vi "Inatke Controller.vi"(8 "error in":errorcluster) -> ()   [LabVIEW 2023]
doc: "This VI executes continuously carrying out the current operation and responding to updates or new operations. It will often contain the timing or control code that is difficult to place directly in TeleOp. This VI generally opens all sensors and motors and isolates the rest of the robot code from knowing how the operations are carried out."
uses:
  <vilib>/Rock Robotics/WPI/Framework/Completion Status.ctl
  Inatke Setpoints.ctl
  <vilib>/Rock Robotics/WPI/Solenoid/WPI_SolenoidValue.ctl
  Transfer/Implementation/Transfer Setpoints.ctl
  Transfer/Implementation/Transfer Operations.ctl
  <vilib>/Rock Robotics/WPI/Solenoid/WPI_SolenoidSetEnum.vi
  Framework/Robot Global Data.vi
  <vilib>/Rock Robotics/Network Tables/NT Write Boolean.vi
panel:
  in  "Bottom":dbl=0.62 format="%#_13g"
  in  "top":dbl=0.52 format="%#_13g"
  in  "Interactive Values":T1
  out "Current\nCmd":string="Started at  09:43:49.164\nDefault: Reserve,  "
  in  "Buttons":cluster{"Execute Cmd":bool, "Abort Cmd":bool}
  out "Command Timing":cluster{"Start Time (ms)":u32, "Iterations":i32}={"Start Time (ms)"=7327, "Iterations"=0}
  out "Status":T2
  # "Tip: It may be helpful to observe inputs and sensor values.\nYou may also want to display tuning or debugging controls."
  # "Interactive Command: You may fill in the settings for a command\nand schedule it with the Execute button. You can observe and abort\nany command while fine tuning the code for the controller."
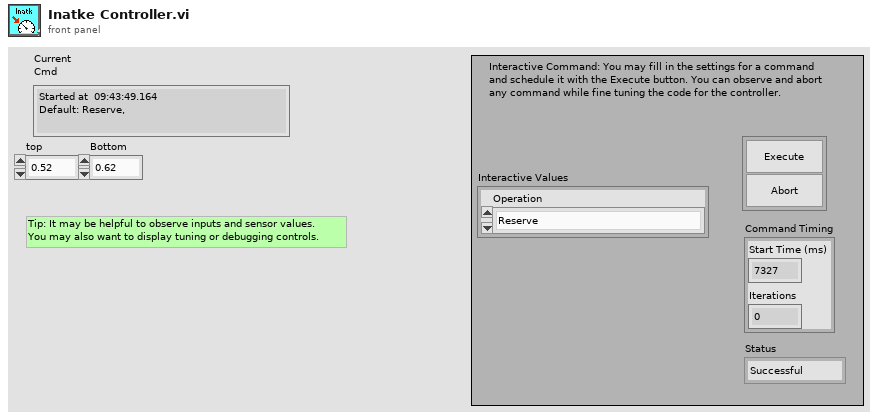
[diagram p1: front panel]
types:
  T1 = typedef "Inatke Setpoints.ctl" = cluster{"Operation":enum16{"Reserve", "Read Current", "Immediate", "Extend", "Retract", "Move Slow", "Reject"}}
  T2 = typedef "Completion Status.ctl" = enum16{"Successful", "Aborted", "Incomplete"}
  T3 = typedef "Command Status Info.ctl" = cluster{"Name":string, "Status":T2, "notifier out":T4}
  T4 = typedef "Completion Notifier.ctl" = refnum<notifier>
  T5 = cluster{"Current Command":T1, "Command Timing":cluster{"Start Time (ms)":u32, "Iterations":i32}, "Command Arguments":cluster{"Command Info":T3, "Description":string, "Default Command":T1, "queue out":refnum<queue>, "Subsystem Name":string}}
  T6 = typedef "WPI_SolenoidValue.ctl" = enum16{"Off", "On", "Forward", "Reverse"}
  T7 = typedef "Transfer Setpoints.ctl" = cluster{"Operation":T8}
  T8 = typedef "Transfer Operations.ctl" = enum16{"Reserve", "Read Current", "Immediate", "On", "Off", "Reject"}
  T9 = enum16{"Reserve", "Read Current", "Immediate", "Extend", "Retract", "Move Slow", "Reject"}
  T10 = typedef "WPI_MotorControlDeviceRef.ctl" = cluster{"DeviceStatus":errorcluster, "Type":T11, "PWM":cluster{"PWM Channel":T12, "DeadBand":T13}, "CAN":cluster{"Device Number":u8, "SetOutput VI Ref":variant, "GetOutput VI Ref":variant, "Enable VI Ref":variant, "Disable VI Ref":variant, "Data":variant}, "Invert":bool, "DIO PWM":cluster{"PWM \"Enable\" Channel":T12, "DIOChannel":T14, "PWM Rate":dbl}}
  T11 = typedef "WPI_MotorControlType.ctl" = enum16{"PWM", "CAN", "DIO PWM"}
  T12 = typedef "FPGA_DIOPWMChannel.ctl" = enum8{"PWM 0", "PWM 1", "PWM 2", "PWM 3", "PWM 4", "PWM 5", "PWM 6", "PWM 7", "PWM 8", "PWM 9", "PWM MXP 0", "PWM MXP 1", "PWM MXP 2", "PWM MXP 3", "PWM MXP 4", "PWM MXP 5", "PWM MXP 6", "PWM MXP 7", "PWM MXP 8", "PWM MXP 9", "Invalid"}
  T13 = typedef "WPI_PWMDeadband.ctl" = cluster{"Name":string, "maxPositivePwm":i32, "minPositivePwm":i32, "centerPwm":i32, "maxNegativePwm":i32, "minNegativePwm":i32, "angularRange":u16}
  T14 = typedef "FPGA_DIOChannel.ctl" = enum8{"DIO 0", "DIO 1", "DIO 2", "DIO 3", "DIO 4", "DIO 5", "DIO 6", "DIO 7", "DIO 8", "DIO 9", "DIO MXP 0", "DIO MXP 1", "DIO MXP 2", "DIO MXP 3", "DIO MXP 4", "DIO MXP 5", "DIO MXP 6", "DIO MXP 7", "DIO MXP 8", "DIO MXP 9", "DIO MXP 10", "DIO MXP 11", "DIO MXP 12", "DIO MXP 13", "DIO MXP 14", "DIO MXP 15", "SPI Port CS1", "SPI Port CS2", "SPI Port CS3", "SPI Port MISO", "SPI Port MOSI", "Invalid"}
  T15 = typedef "WPI_SolenoidDevRef.ctl" = cluster{"DevStatus":errorcluster, "Pneumatics Control Module":u8, "Forward Solenoid Channel":T16, "Reverse Solenoid Channel":T16}
  T16 = typedef "WPI_SolenoidChannel.ctl" = enum8{"Solenoid 0", "Solenoid 1", "Solenoid 2", "Solenoid 3", "Solenoid 4", "Solenoid 5", "Solenoid 6", "Solenoid 7", "Solenoid 8", "Solenoid 9", "Solenoid 10", "Solenoid 11", "Solenoid 12", "Solenoid 13", "Solenoid 14", "Solenoid 15", "Invalid"}
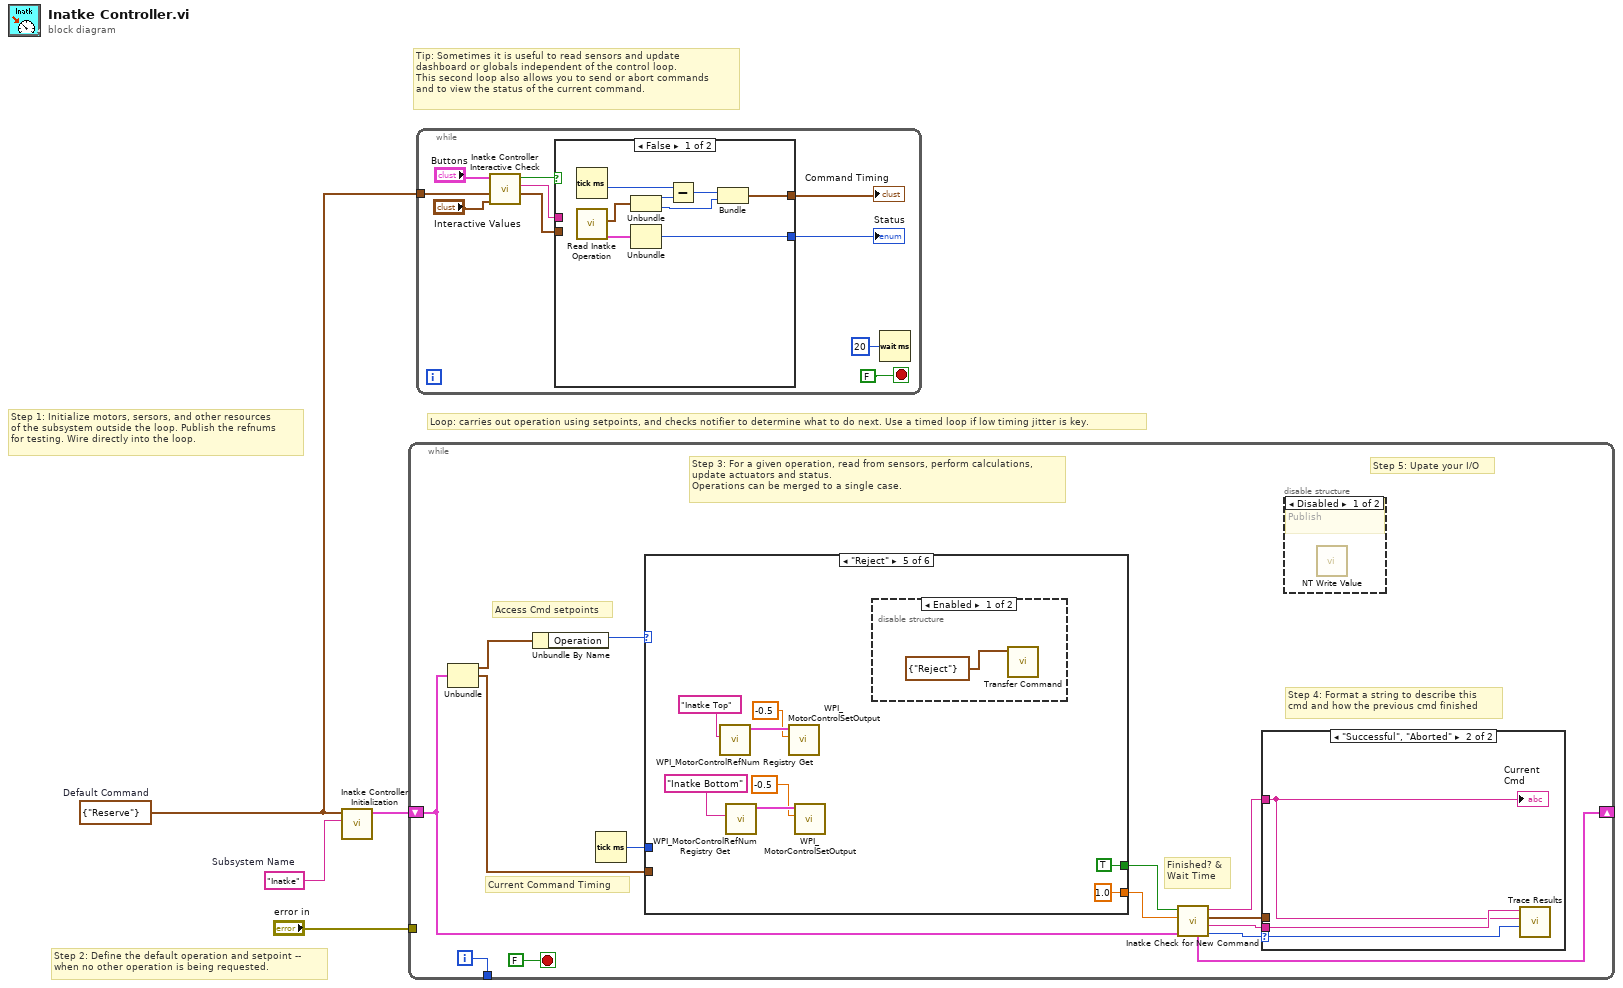
[diagram p0: block diagram]
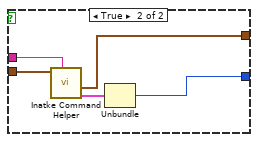
[diagram p2: hidden frame]
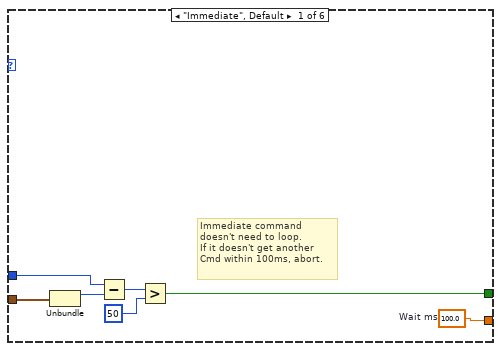
[diagram p5: hidden frame]
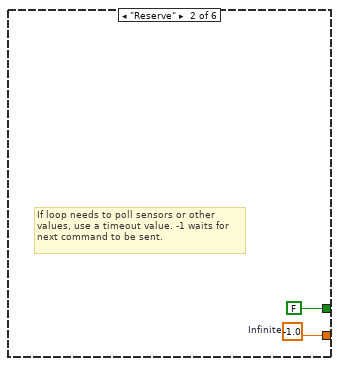
[diagram p6: hidden frame]
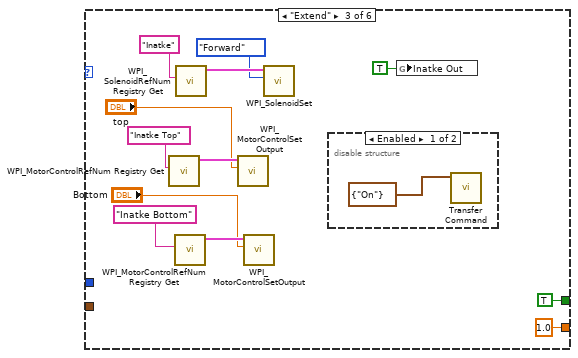
[diagram p7: hidden frame]
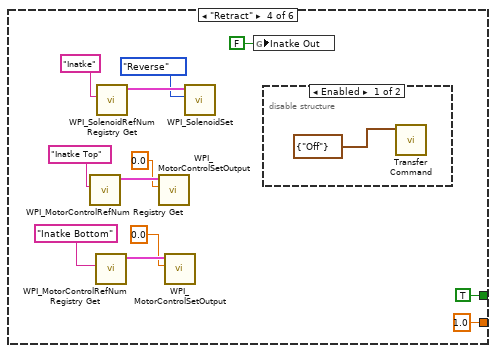
[diagram p9: hidden frame]
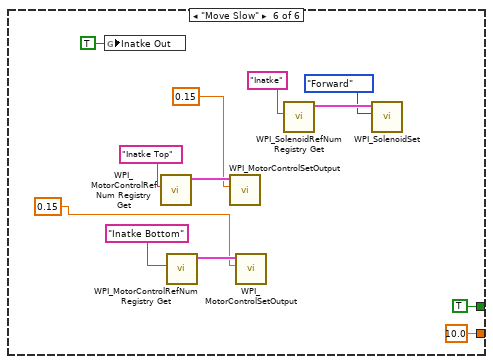
[diagram p12: hidden frame]
diagram:
  w1 = T1 {"Operation"=enum."Reserve"}  # Default Command
  w2 = "Inatke"  # Subsystem Name
  # "Tip: Sometimes it is useful to read sensors and update\ndashboard or globals independent of the control loop.\nThis second loop also allows you to send or abort commands\nand to view the status of the current command."
  # "Step 2: Define the default operation and setpoint --\nwhen no other operation is being requested."
  # "Step 1: Initialize motors, sersors, and other resources\nof the subsystem outside the loop. Publish the refnums\nfor testing. Wire directly into the loop."
  # "Loop: carries out operation using setpoints, and checks notifier to determine what to do next. Use a timed loop if low timing jitter is key."
  n1 = call "Inatke Controller Initialization.vi"("Subsystem Name"=w2, "Default Command"=w1) -> ("Current Command"=w3:T5)  [unwired: 9 in]
  n2 = while {
    shift-right: [w12] -> _
    shift-left: w3 -> [w5]
    tunnel: [w17] -> _
    tunnel: "error in" -> [_]
    i -> [w17]
    stop <- FALSE stop-if-true
    # "Step 5: Upate your I/O"
    # "Step 4: Format a string to describe this\ncmd and how the previous cmd finished"
    # "Current Command Timing"
    # "Access Cmd setpoints"
    # "Finished? &\nWait Time"
    # "Step 3: For a given operation, read from sensors, perform calculations,\nupdate actuators and status.\nOperations can be merged to a single case."
    n3 = Unbundle(w5) -> ("Current Command"=w16:T1, "Command Timing"=w13:cluster{"Start Time (ms)":u32, "Iterations":i32})  [unwired: 1 out]
    n4 = Unbundle By Name(w16) -> ("Operation"=w15:T9)
    n5 = Tick Count (ms)() -> (millisecond timer value=w14:u32)
    n6 = case shown="\"Reject\"" w15 {
      tunnel: [w28 w30 1.0 ("Infinite") 1.0 ("Infinite") 1.0 ("Infinite") 10.0 ("Infinite")] -> w10
      tunnel: [w22 FALSE ("ignore previous (F)") TRUE ("ignore previous (F)") TRUE ("ignore previous (F)") TRUE ("ignore previous (F)") TRUE ("ignore previous (F)")] -> w11
      tunnel: w13 -> [w24 _ _ _ _ _]
      tunnel: w14 -> [w23 _ _ _ _ _]
      frame "Immediate", Default {
        w28 = 100.0  # Wait ms
        # "Immediate command\ndoesn't need to loop.\nIf it doesn't get another\nCmd within 100ms, abort."
        n7 = Unbundle(w24) -> ("Start Time (ms)"=w27:u32)  [unwired: 1 out]
        n8 = Subtract(x=w23, y=w27) -> (x-y=w26:u32)
        n9 = Greater?(x=w26, y=u8 50 ("Left Motor")) -> (0:w22:bool)
      }
      frame "Reserve" {
        w30 = -1.0  # Infinite
        # "If loop needs to poll sensors or other\nvalues, use a timeout value. -1 waits for\nnext command to be sent."
      }
      frame "Extend" {
        n10 = call <vilib>:"WPI_MotorControlRefNum Registry Get.vi"("refnum name"="Inatke Top") -> ("MotorControlDevRef"=w38:T10)  [unwired: 9 in, 1 out]
        n11 = call <vilib>:"WPI_MotorControlRefNum Registry Get.vi"("refnum name"="Inatke Bottom") -> ("MotorControlDevRef"=w35:T10)  [unwired: 9 in, 1 out]
        n12 = call <vilib>:"WPI_SolenoidRefNum Registry Get.vi"("refnum name"="Inatke") -> ("SolenoidDevRef"=w42:T15)  [unwired: 9 in, 1 out]
        n13 = call <vilib>:"WPI_MotorControlSetOutput.vi"("Output"="top", "MotorControlDevRef"=w38) -> ()  [unwired: 7 in, 3 out]
        n14 = call <vilib>:"WPI_MotorControlSetOutput.vi"("Output"="Bottom", "MotorControlDevRef"=w35) -> ()  [unwired: 7 in, 3 out]
        n15 = call-poly <vilib>:"WPI_SolenoidSet.vi"("Value"=WPI_SolenoidValue."Forward", "SolenoidDevRef"=w42) -> ()  [unwired: 8 in, 2 out]
        n16 = disable-structure shown="Enabled" {
          frame Enabled {
            n17 = call "Transfer Command.vi"("SubSystem Data"=T7 {"Operation"=enum."On"}) -> ()  [unwired: 10 in, 1 out]
          }
          frame Disabled {
          }
        }
        n18 = global write "Robot Global Data.vi" "Inatke Out"(TRUE ("Inatke Out")) -> ()
      }
      frame "Retract" {
        n19 = call <vilib>:"WPI_MotorControlRefNum Registry Get.vi"("refnum name"="Inatke Top") -> ("MotorControlDevRef"=w51:T10)  [unwired: 9 in, 1 out]
        n20 = call <vilib>:"WPI_MotorControlRefNum Registry Get.vi"("refnum name"="Inatke Bottom") -> ("MotorControlDevRef"=w48:T10)  [unwired: 9 in, 1 out]
        n21 = call <vilib>:"WPI_SolenoidRefNum Registry Get.vi"("refnum name"="Inatke") -> ("SolenoidDevRef"=w55:T15)  [unwired: 9 in, 1 out]
        n22 = call <vilib>:"WPI_MotorControlSetOutput.vi"("Output"=0.0, "MotorControlDevRef"=w51) -> ()  [unwired: 7 in, 3 out]
        n23 = call <vilib>:"WPI_MotorControlSetOutput.vi"("Output"=0.0, "MotorControlDevRef"=w48) -> ()  [unwired: 7 in, 3 out]
        n24 = call-poly <vilib>:"WPI_SolenoidSet.vi"("Value"=WPI_SolenoidValue."Reverse", "SolenoidDevRef"=w55) -> ()  [unwired: 8 in, 2 out]
        n25 = global write "Robot Global Data.vi" "Inatke Out"(FALSE ("Inatke Out")) -> ()
        n26 = disable-structure shown="Enabled" {
          frame Enabled {
            n27 = call "Transfer Command.vi"("SubSystem Data"=T7 {"Operation"=enum."Off"}) -> ()  [unwired: 10 in, 1 out]
          }
          frame Disabled {
          }
        }
      }
      frame "Reject" {
        n28 = call <vilib>:"WPI_MotorControlRefNum Registry Get.vi"("refnum name"="Inatke Top") -> ("MotorControlDevRef"=w63:T10)  [unwired: 9 in, 1 out]
        n29 = call <vilib>:"WPI_MotorControlRefNum Registry Get.vi"("refnum name"="Inatke Bottom") -> ("MotorControlDevRef"=w60:T10)  [unwired: 9 in, 1 out]
        n30 = call <vilib>:"WPI_MotorControlSetOutput.vi"("Output"=-0.5, "MotorControlDevRef"=w63) -> ()  [unwired: 7 in, 3 out]
        n31 = call <vilib>:"WPI_MotorControlSetOutput.vi"("Output"=-0.5, "MotorControlDevRef"=w60) -> ()  [unwired: 7 in, 3 out]
        n32 = disable-structure shown="Enabled" {
          frame Enabled {
            n33 = call "Transfer Command.vi"("SubSystem Data"=T7 {"Operation"=enum."Reject"}) -> ()  [unwired: 10 in, 1 out]
          }
          frame Disabled {
          }
        }
      }
      frame "Move Slow" {
        n34 = global write "Robot Global Data.vi" "Inatke Out"(TRUE ("Inatke Out")) -> ()
        n35 = call <vilib>:"WPI_MotorControlRefNum Registry Get.vi"("refnum name"="Inatke Top") -> ("MotorControlDevRef"=w76:T10)  [unwired: 9 in, 1 out]
        n36 = call <vilib>:"WPI_MotorControlRefNum Registry Get.vi"("refnum name"="Inatke Bottom") -> ("MotorControlDevRef"=w75:T10)  [unwired: 9 in, 1 out]
        n37 = call <vilib>:"WPI_MotorControlSetOutput.vi"("Output"=0.15, "MotorControlDevRef"=w76) -> ()  [unwired: 7 in, 3 out]
        n38 = call <vilib>:"WPI_MotorControlSetOutput.vi"("Output"=0.15, "MotorControlDevRef"=w75) -> ()  [unwired: 7 in, 3 out]
        n39 = call <vilib>:"WPI_SolenoidRefNum Registry Get.vi"("refnum name"="Inatke") -> ("SolenoidDevRef"=w69:T15)  [unwired: 9 in, 1 out]
        n40 = call-poly <vilib>:"WPI_SolenoidSet.vi"("Value"=WPI_SolenoidValue."Forward", "SolenoidDevRef"=w69) -> ()  [unwired: 8 in, 2 out]
      }
    }
    n41 = call "Inatke Check for New Command.vi"("Current Command"=w5, "Wait time (ms)"=w10, "Finished?"=w11) -> ("Completion"=w6:T2, "Subsystem Name"=w7:string, "Current Command"=w8:T1, "Initial Trace String"=w9:string, "NextCommand"=w12:T5)  [unwired: 4 in]
    n42 = case shown="\"Successful\", \"Aborted\"" w6 {
      selector: w6 -> [_ w21]
      tunnel: w9 -> [_ w19]
      tunnel: w8 -> [_ _]
      tunnel: w7 -> [_ w20]
      frame "Incomplete", Default {
        # "Continuing current command"
      }
      frame "Successful", "Aborted" {
        # "Report and setup for next command"
        n43 = call <vilib>:"Trace Results.vi"("Status of previous command"=w21, "Description"=w19, "Subsystem"=w20) -> ()  [unwired: 9 in]
        "Current\nCmd" <- w19
      }
    }
    n44 = disable-structure shown="Disabled" {
      frame Disabled {
        # "Publish"
        n45 = call-poly <vilib>:"NT Write Value.vi"() -> ()  [unwired: 11 in, 1 out]
      }
      frame Enabled {
      }
    }
  }
  n46 = while {
    tunnel: w1 -> [w84]
    stop <- FALSE stop-if-true
    n47 = call "Inatke Controller Interactive Check.vi"("Interactive Command in"="Interactive Values", "Default Command"=w84, "Buttons"="Buttons") -> ("Interactive Command out"=w81:T1, "Trace String"=w82:string, "Schedule"=w83:bool)  [unwired: 6 in]
    n48 = case shown="False" w83 {
      tunnel: [w95 w100] -> w80
      tunnel: w81 -> [_ w98]
      tunnel: [w90 w96] -> w79
      tunnel: w82 -> [_ w99]
      frame False {
        n49 = Tick Count (ms)() -> (millisecond timer value=w92:u32)
        n50 = call "Read Inatke Operation.vi"() -> ("Command Info"=w91:T3, "Command Timing"=w89:cluster{"Start Time (ms)":u32, "Iterations":i32})  [unwired: 9 in, 1 out]
        n51 = Unbundle(w89) -> ("Start Time (ms)"=w94:u32, "Iterations"=w88:i32)
        n52 = Unbundle(w91) -> ("Status"=w95:T2)  [unwired: 2 out]
        n53 = Subtract(x=w92, y=w94) -> (x-y=w93:u32)
        n54 = Bundle(w93, "Iterations"=w88) -> (w90:cluster{u32, "Iterations":i32})  [unwired: 1 in]
      }
      frame True {
        n55 = call "Inatke Command Helper.vi"("Description"=w99, "SubSystem Data"=w98) -> ("Command Info Out"=w97:T3, "Command Timing"=w96:cluster{"Start Time (ms)":u32, "Iterations":i32})  [unwired: 7 in, 1 out]
        n56 = Unbundle(w97) -> ("Status"=w100:T2)  [unwired: 2 out]
      }
    }
    "Status" <- w80
    "Command Timing" <- w79
    n57 = Wait (ms)(milliseconds to wait=u32 20) -> ()  [unwired: 1 out]
  }
